vi "Create.vi"(0 "array of point offsets":T1[](array[typedef]), 11 "error in":errorcluster) -> (4 "eye scan point iterator out":refnum<class "niHighSpeedSerial N Point Eye Scan Point Iterator v1 Host.lvclass">, 15 "error out":errorcluster)   [LabVIEW 2014, in "niHighSpeedSerial N Point Eye Scan Point Iterator v1 Host.lvclass"]
doc: "Creates a Point Iterator object.\n\n<B>Input Parameters</B>\n\n<B>array of point offsets</B> is the array of point offsets to measure using Eye Scan.\n\n<B>array of point offsets.horizontal offset</B> is the horizontal offset of the point.\n\n<B>array of point offsets.vertical offset</B> is the vertical offset of the point\n\n<B>error in</B> describes error conditions that occur before this node runs. This input provides standard 'error in' functionality.\n\n<B>Output Parameters</B>\n\n<B>eye scan point iterator out</B> is the outgoing wire for the Eye Scan Point Iterator class object\n\n<B>error out</B> contains error information. This output provides standard 'error out' functionality."
uses:
  <instrlib>/niHighSpeedSerial/Eye Scan/v1/Host/Impl/N Pt Iter/niHighSpeedSerial N Point Eye Scan Point Iterator v1 Host.lvclass
  <instrlib>/niHighSpeedSerial/Eye Scan/v1/Host/Common/Public/Point Offsets.ctl
  <instrlib>/niHighSpeedSerial/Eye Scan/v1/Host/Common/Public/Point.ctl
  <instrlib>/niHighSpeedSerial/Eye Scan/v1/Host/Impl/N Pt Iter/niHighSpeedSerial N Point Eye Scan Point Iterator v1 Host.lvclass/niHighSpeedSerial N Point Eye Scan Point Iterator v1 Host.ctl
  <instrlib>/niHighSpeedSerial/Eye Scan/v1/Host/Common/niHighSpeedSerial Eye Scan Common v1 Host.lvlib
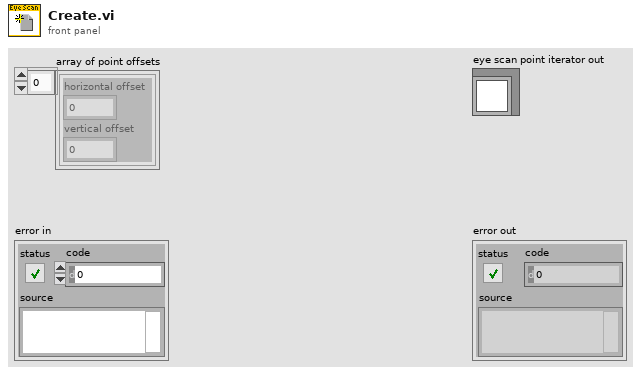
[diagram p1: front panel]
types:
  T1 = typedef "niHighSpeedSerial Eye Scan Common v1 Host.lvlib/Point Offsets.ctl" = cluster{"horizontal offset":i16, "vertical offset":i8}
  T2 = typedef "niHighSpeedSerial Eye Scan Common v1 Host.lvlib/Point.ctl" = cluster{"point offsets":T1, "sample count":u64, "error count":u64, "bit error ratio":dbl}
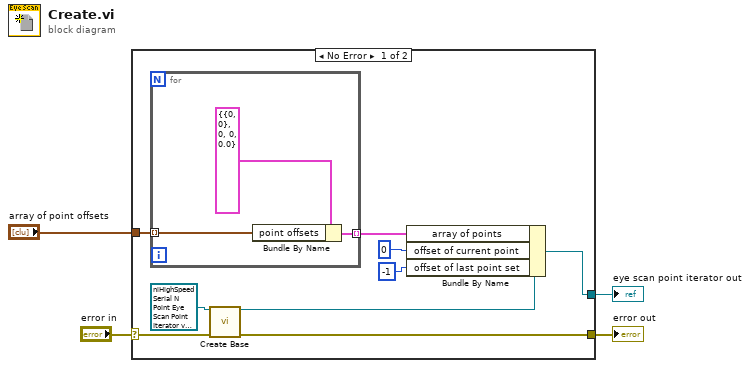
[diagram p0: block diagram]
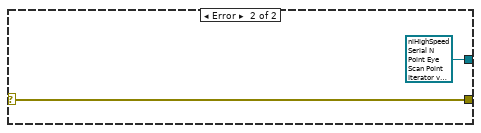
[diagram p2: hidden frame]
diagram:
  n1 = case shown="No Error" "error in" {
    selector: "error in" -> [w10 w18]
    tunnel: [w12 w18] -> w3
    tunnel: [w13 refnum<class "niHighSpeedSerial N Point Eye Scan Point Iterator v1 Host.lvclass"> refnum ("N Point Eye Scan Point Iterator.lvclass")] -> w2
    tunnel: "array of point offsets" -> [w11 _]
    frame No Error {
      n2 = for {
        tunnel: w11 -> [w16] mode=indexing
        tunnel: [w15] -> w7 mode=indexing
        n3 = Bundle By Name(cluster=T2 {"point offsets"={"horizontal offset"=0, "vertical offset"=0}, "sample count"=0, "error count"=0, "bit error ratio"=0.0} ("point"), "point offsets"=w16) -> (w15:T2)
      }
      n4 = call-dynamic "Create Base.vi"("eye scan point iterator"=refnum<class "niHighSpeedSerial N Point Eye Scan Point Iterator v1 Host.lvclass"> refnum ("N Point Eye Scan Point Iterator.lvclass"), "error in"=w10) -> ("eye scan point iterator out"=w8:refnum<class "niHighSpeedSerial N Point Eye Scan Point Iterator v1 Host.lvclass">, "error out"=w12:errorcluster)  [unwired: 12 in]
      n5 = Bundle By Name(cluster=w8, "array of points"=w7, "offset of current point"=0 ("Current Point Offset In Array"), "offset of last point set"=-1) -> (w13:refnum<class "niHighSpeedSerial N Point Eye Scan Point Iterator v1 Host.lvclass">)
    }
    frame Error {
    }
  }
  "eye scan point iterator out" <- w2
  "error out" <- w3
